vi "Pre Launch Init.vi"(11 "SM EOL Station Actor in":refnum<class "OPC Server.lvclass">) -> (0 "error out":errorcluster, 3 "SM EOL Station Actor out":refnum<class "OPC Server.lvclass">)   [LabVIEW 2021, in "OPC Server.lvlib" / "OPC Server.lvclass"]
doc: "(<B>Filename</B>: Actor Framework.lvlib:Actor.lvclass:Pre Launch Init.vi)\n\nDefines behavior that occurs after the Launch Nested Actor method is invoked but before the actor's Actor Core method begins running.\n\nBy default, this method does nothing. A descendant class may override it to define behavior."
uses:
  OPC Server.lvclass
  OPC Server.lvclass/OPC Server.ctl
  <vilib>/ActorFramework/Actor/Actor.lvclass
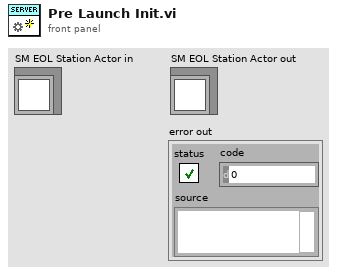
[diagram p1: front panel]
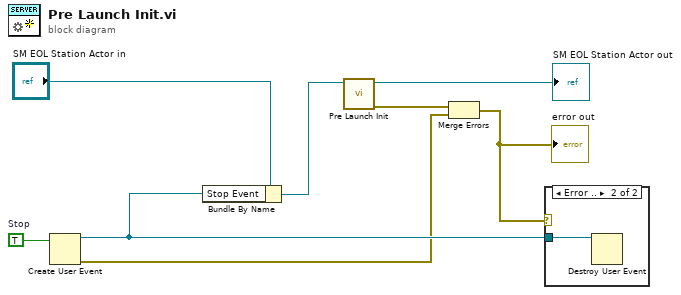
[diagram p0: block diagram]
diagram:
  w8 = TRUE  # Stop
  n1 = Create User Event(user event datatype=w8) -> (user event=w6:refnum<user-event>, error out=w5:errorcluster)  [unwired: 1 in]
  n2 = Bundle By Name(cluster="SM EOL Station Actor in", "Stop Event"=w6) -> (w4:refnum<class "OPC Server.lvclass">)
  n3 = call-parent "Pre Launch Init.vi"("Actor in"=w4) -> ("error out"=w2:errorcluster, "Actor out"=→"SM EOL Station Actor out":refnum<class "OPC Server.lvclass">)  [unwired: 9 in]
  n4 = Merge Errors(w2, w5) -> (w3:errorcluster)
  "error out" <- w3
  n5 = case shown="Error .." w3 {
    tunnel: w6 -> [_ w9]
    frame No Error {
    }
    frame Error {
      n6 = Destroy User Event(user event=w9) -> ()  [unwired: 1 in, 1 out]
    }
  }
